vi "subviTOTHDAVIDANDREI633AB.vi"(8 "error in (no error)":errorcluster, 11 "Array":dbl[](array[numeric])) -> (0 "error out":errorcluster, 3 "Outputs":dbl[](array[numeric]))   [LabVIEW 2024]
uses:
  <vilib>/National Instruments/NI Super Simple Neural Networks/Types/Teaching Settings.ctl
  <vilib>/National Instruments/NI Super Simple Neural Networks/Types/Error Evaluation.ctl
  <vilib>/National Instruments/NI Super Simple Neural Networks/API/Create 1 Hidden Layer.vi
  <vilib>/National Instruments/NI Super Simple Neural Networks/Neural Network.lvclass
panel:
  in  "stop":bool
  in  "Path":path
  out "Error Trend Out":dbl[](array[numeric])
  out "Teaching Time (s)":dbl
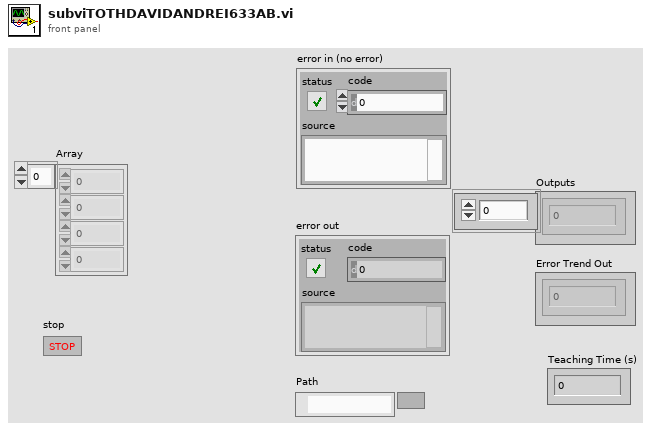
[diagram p1: front panel]
types:
  T1 = typedef "Neural Network.lvclass/Teaching Settings.ctl" = cluster{"Max Epocs":u64, "Error Goal":dbl, "Max Time (s)":dbl, "Error Evaluation":T2, "# Vectors per Iteration":i32}
  T2 = typedef "Neural Network.lvclass/Error Evaluation.ctl" = enum16{"Over Both Sets", "Over Validation Set", "Over Teaching Set"}
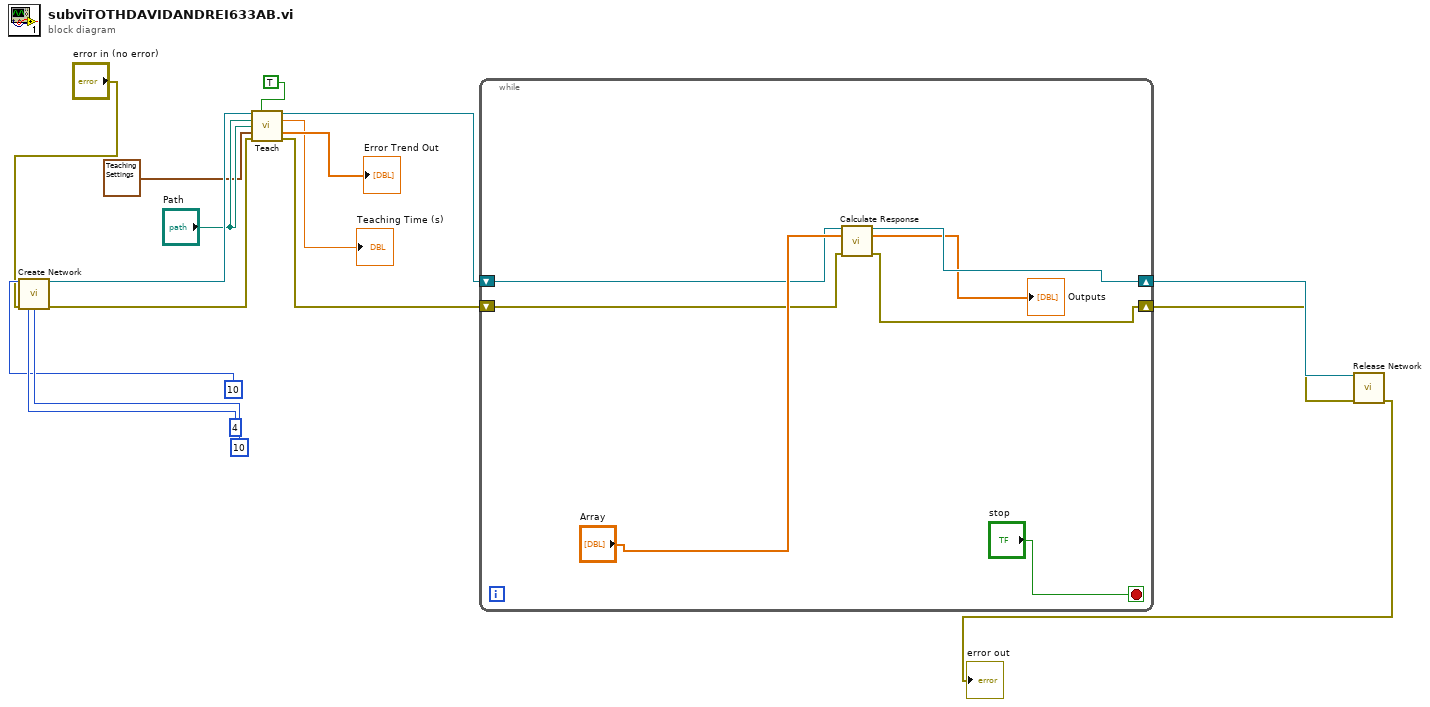
[diagram p0: block diagram]
diagram:
  n1 = call-poly <vilib>:"Create Network.vi"("1st Hidden Layer Neurons"=u32 10, "Error In"="error in (no error)", "# Inputs"=u32 4, "Output Neurons/Outputs"=u32 10) -> ("Neural Network Out"=w10:refnum<class "Neural Network.lvclass">, "Error Out"=w6:errorcluster)  [unwired: 10 in]
  n2 = call <vilib>:"Teach.vi"("Neural Network In"=w10, "Enable Growing/Prunning"=TRUE, "Teaching Set Path In"="Path", "Validation Set Path In"="Path", "Settings In"=T1 {"Max Epocs"=10000, "Error Goal"=10.0, "Max Time (s)"=10.0, "Error Evaluation"=enum."Over Teaching Set", "# Vectors per Iteration"=200}, "Error In"=w6) -> ("Neural Network Out"=w4:refnum<class "Neural Network.lvclass">, "Teaching Time (s)"=→"Teaching Time (s)":dbl, "Error Trend Out"=→"Error Trend Out":dbl[], "Error Out"=w5:errorcluster)  [unwired: 5 in, 1 out]
  n3 = while {
    shift-right: [w22] -> w12
    shift-left: w4 -> [w18]
    shift-right: [w21] -> w11
    shift-left: w5 -> [w17]
    stop <- "stop" stop-if-true
    n4 = call <vilib>:"Calculate Response.vi"("Neural Network In"=w18, "Inputs"="Array", "Error In"=w17) -> ("Neural Network Out"=w22:refnum<class "Neural Network.lvclass">, "Outputs"=→"Outputs":dbl[], "Error Out"=w21:errorcluster)  [unwired: 10 in]
  }
  n5 = call <vilib>:"Release Network.vi"("Neural Network"=w12, "Error In"=w11) -> ("Error Out"=→"error out":errorcluster)  [unwired: 13 in]
